vi "Overlay.vi"(0 "Image":T2, 5 "FullArray":dbl[][](array[numeric]), 7 "SelectedGoalSubarray":dbl[](array[numeric]), 9 "ProjectedPosition":cluster{dbl, dbl}, 11 "Enabled Overlay":T1, 13 "encoder":dbl) -> (4 "ImageOut":T2(plugin-control))   [LabVIEW 2012]
uses:
  <vilib>/vision/Image Controls.llb/IMAQ Image.ctl
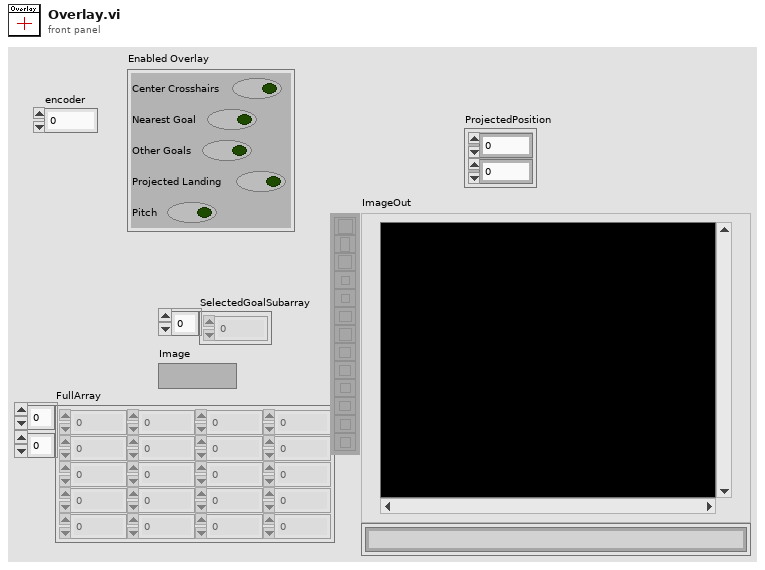
[diagram p1: front panel]
types:
  T1 = cluster{"Center Crosshairs":bool, "Nearest Goal":bool, "Other Goals":bool, "Projected Landing":bool, "Pitch":bool}
  T2 = typedef "IMAQ Image.ctl" = refnum<image>
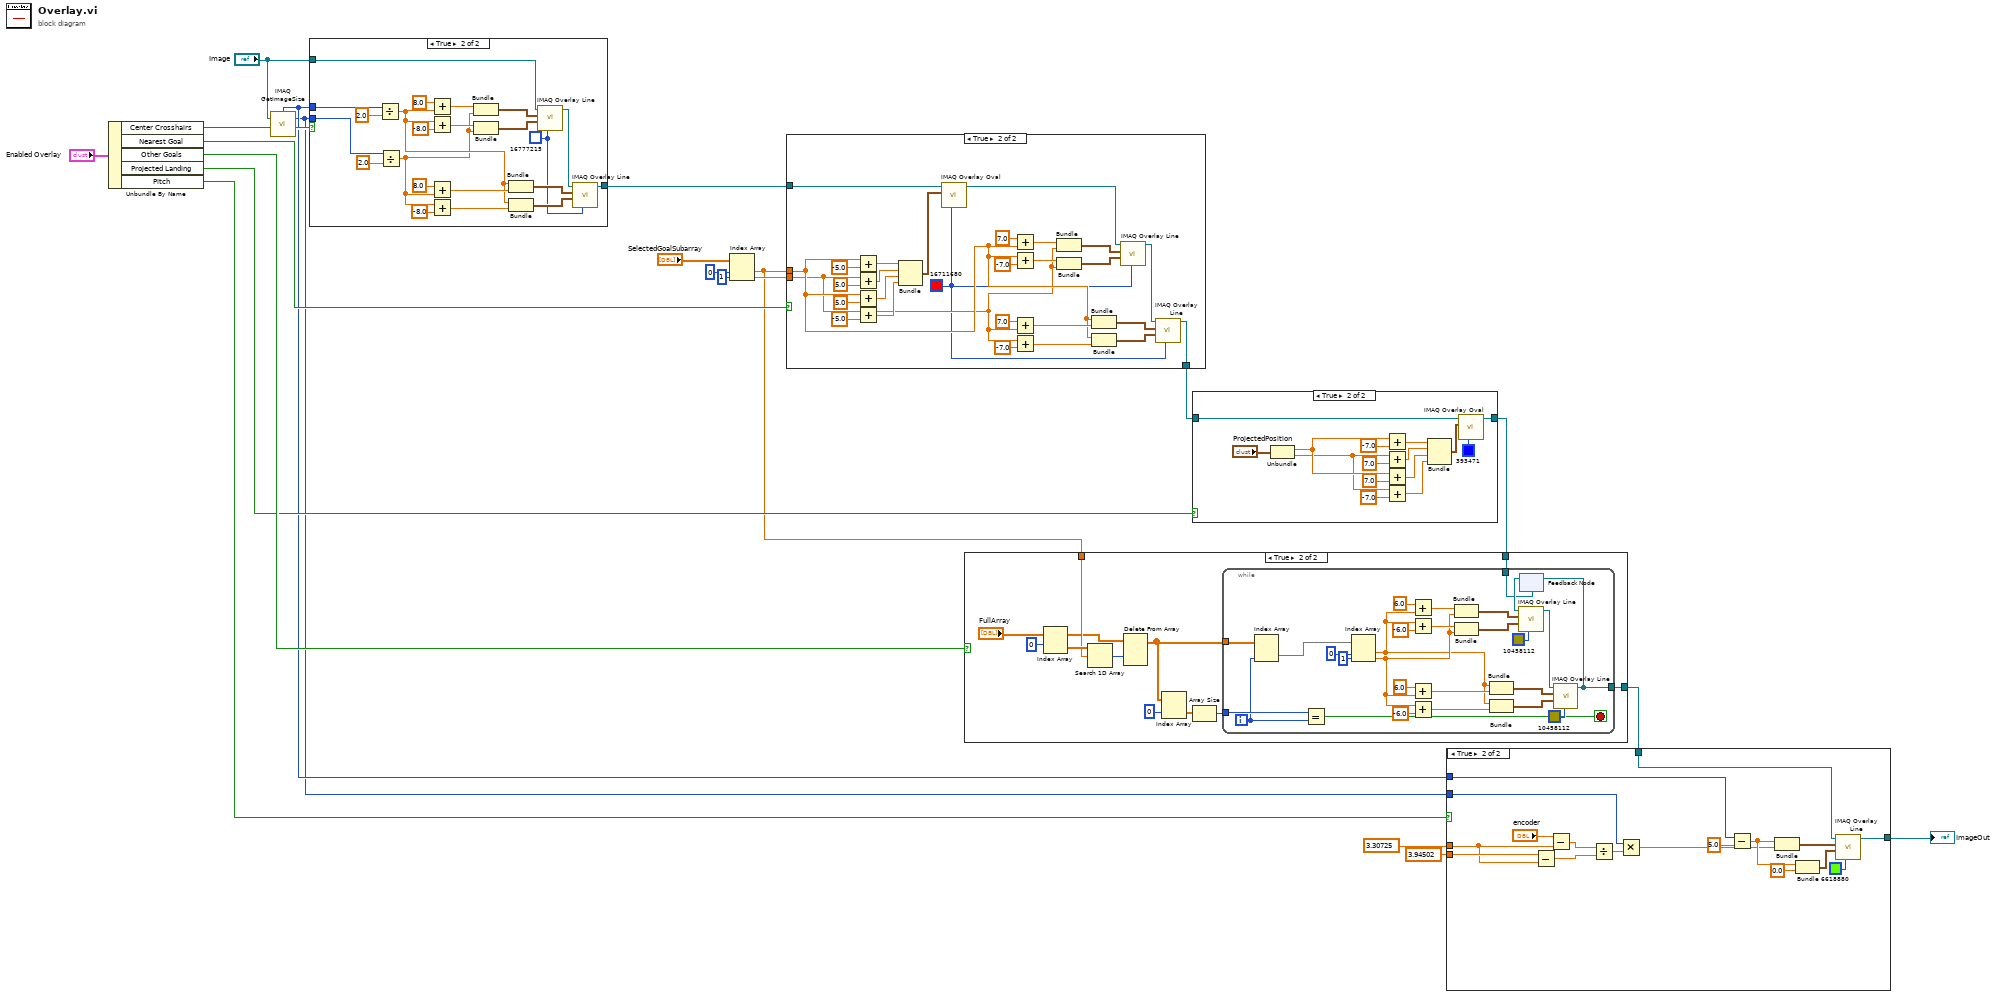
[diagram p0: block diagram]
diagram:
  n1 = Unbundle By Name("Enabled Overlay") -> ("Center Crosshairs"=w15:bool, "Nearest Goal"=w14:bool, "Other Goals"=w13:bool, "Projected Landing"=w12:bool, "Pitch"=w3:bool)
  n2 = call "IMAQ GetImageSize"("Image"="Image") -> ("Y Resolution"=w5:i32, "X Resolution"=w6:i32)  [unwired: 3 in, 1 out]
  n3 = case shown="True" w15 {
    tunnel: [w22 w27] -> w16
    tunnel: "Image" -> [w22 w25]
    tunnel: w5 -> [_ w24]
    tunnel: w6 -> [_ w23]
    frame False {
    }
    frame True {
      w26 = u32 16777215 ("Color")
      n4 = Divide(x=w23, y=2.0) -> (x/y=w29:dbl)
      n5 = Divide(x=w24, y=2.0) -> (x/y=w28:dbl)
      n6 = Add(x=8.0, y=w29) -> (x+y=w39:dbl)
      n7 = Add(x=w29, y=-8.0) -> (x+y=w40:dbl)
      n8 = Add(x=8.0, y=w28) -> (x+y=w34:dbl)
      n9 = Add(x=w28, y=-8.0) -> (x+y=w33:dbl)
      n10 = Bundle(w39, w28) -> (w38:cluster{dbl, dbl})  [unwired: 1 in]
      n11 = Bundle(w40, w28) -> (w37:cluster{dbl, dbl})  [unwired: 1 in]
      n12 = Bundle(w29, w34) -> (w36:cluster{dbl, dbl})  [unwired: 1 in]
      n13 = Bundle(w29, w33) -> (w35:cluster{dbl, dbl})  [unwired: 1 in]
      n14 = call "IMAQ Overlay Line"("Color"=w26, "End Point"=w37, "Start Point"=w38, "Image"=w25) -> ("Image Out"=w32:T2)  [unwired: 6 in, 1 out]
      n15 = call "IMAQ Overlay Line"("Color"=w26, "End Point"=w35, "Start Point"=w36, "Image"=w32) -> ("Image Out"=w27:T2)  [unwired: 6 in, 1 out]
    }
  }
  n16 = Index Array(array="SelectedGoalSubarray", index #1=0 ("index"), index #2=1 ("index")) -> (element #1=w9:dbl, element #2=w18:dbl)
  n17 = case shown="True" w14 {
    tunnel: w9 -> [_ w51]
    tunnel: w18 -> [_ w50]
    tunnel: [w45 w48] -> w11
    tunnel: w16 -> [w45 w46]
    frame False {
    }
    frame True {
      w47 = u32 16711680 ("Color")
      n18 = Add(x=w51, y=-5.0) -> (x+y=w70:dbl)
      n19 = Add(x=w50, y=5.0) -> (x+y=w71:dbl)
      n20 = Add(x=w51, y=5.0) -> (x+y=w69:dbl)
      n21 = Add(x=w50, y=-5.0) -> (x+y=w66:dbl)
      n22 = Bundle(w70, w71, w69, w66) -> (w65:cluster{dbl, dbl, dbl, dbl})  [unwired: 1 in]
      n23 = call "IMAQ Overlay Oval"("Color"=w47, "Bounding Rectangle"=w65, "Image"=w46) -> ("Image Out"=w49:T2)  [unwired: 7 in, 1 out]
      n24 = Add(x=7.0, y=w51) -> (x+y=w59:dbl)
      n25 = Add(x=w51, y=-7.0) -> (x+y=w60:dbl)
      n26 = Add(x=7.0, y=w50) -> (x+y=w54:dbl)
      n27 = Add(x=w50, y=-7.0) -> (x+y=w53:dbl)
      n28 = Bundle(w59, "Numeric"=w50) -> (w58:cluster{dbl, "Numeric":dbl})  [unwired: 1 in]
      n29 = Bundle(w60, "Numeric"=w50) -> (w57:cluster{dbl, "Numeric":dbl})  [unwired: 1 in]
      n30 = Bundle("Numeric"=w51, w54) -> (w56:cluster{"Numeric":dbl, dbl})  [unwired: 1 in]
      n31 = Bundle("Numeric"=w51, w53) -> (w55:cluster{"Numeric":dbl, dbl})  [unwired: 1 in]
      n32 = call "IMAQ Overlay Line"("Color"=w47, "End Point"=w57, "Start Point"=w58, "Image"=w49) -> ("Image Out"=w52:T2)  [unwired: 6 in, 1 out]
      n33 = call "IMAQ Overlay Line"("Color"=w47, "End Point"=w55, "Start Point"=w56, "Image"=w52) -> ("Image Out"=w48:T2)  [unwired: 6 in, 1 out]
    }
  }
  n34 = case shown="True" w12 {
    tunnel: [w74 w80] -> w10
    tunnel: w11 -> [w74 w81]
    frame False {
    }
    frame True {
      n35 = Unbundle("ProjectedPosition") -> (w77:dbl, w76:dbl)
      n36 = Add(x=w77, y=-7.0) -> (x+y=w86:dbl)
      n37 = Add(x=w76, y=7.0) -> (x+y=w87:dbl)
      n38 = Add(x=w77, y=7.0) -> (x+y=w85:dbl)
      n39 = Add(x=w76, y=-7.0) -> (x+y=w82:dbl)
      n40 = Bundle(w86, w87, w85, w82) -> (w78:cluster{dbl, dbl, dbl, dbl})  [unwired: 1 in]
      n41 = call "IMAQ Overlay Oval"("Color"=u32 393471, "Bounding Rectangle"=w78, "Image"=w81) -> ("Image Out"=w80:T2)  [unwired: 7 in, 1 out]
    }
  }
  n42 = case shown="True" w13 {
    tunnel: [w90 w99] -> w7
    tunnel: w10 -> [w90 w98]
    tunnel: w9 -> [_ w97]
    frame False {
    }
    frame True {
      n43 = Index Array(array="FullArray", index (row)=0) -> (element=w101:dbl[])  [unwired: 1 in]
      n44 = Search 1D Array(1D array=w101, element=w97) -> (index of element=w96:i32)  [unwired: 1 in]
      n45 = Delete From Array(array="FullArray", index (row)=w96) -> (array with subset deleted=w93:dbl[][])  [unwired: 2 in, 1 out]
      n46 = Index Array(array=w93, index (row)=0) -> (element=w94:dbl[])  [unwired: 1 in]
      n47 = Array Size(array=w94) -> (size(s)=w92:i32)
      n48 = while {
        tunnel: w93 -> [w106]
        tunnel: [w109] -> w99
        tunnel: w98 -> [w107]
        tunnel: w92 -> [w104]
        i -> [w103]
        stop <- w102 stop-if-true
        n49 = Index Array(array=w106, index (col)=w103) -> (element=w105:dbl[])  [unwired: 1 in]
        n50 = Equal?(x=w104, y=w103) -> (x = y?=w102:bool)
        n51 = Index Array(array=w105, index #1=0 ("index"), index #2=1 ("index")) -> (element #1=w111:dbl, element #2=w120:dbl)
        n52 = Add(x=6.0, y=w111) -> (x+y=w121:dbl)
        n53 = Add(x=w111, y=-6.0) -> (x+y=w122:dbl)
        n54 = Add(x=6.0, y=w120) -> (x+y=w114:dbl)
        n55 = Add(x=w120, y=-6.0) -> (x+y=w113:dbl)
        n56 = Bundle(w121, "Numeric"=w120) -> (w119:cluster{dbl, "Numeric":dbl})  [unwired: 1 in]
        n57 = Bundle(w122, "Numeric"=w120) -> (w118:cluster{dbl, "Numeric":dbl})  [unwired: 1 in]
        n58 = Bundle("Numeric"=w111, w114) -> (w116:cluster{"Numeric":dbl, dbl})  [unwired: 1 in]
        n59 = Bundle("Numeric"=w111, w113) -> (w115:cluster{"Numeric":dbl, dbl})  [unwired: 1 in]
        n60 = feedback #1(w107) -> (w110:T2)
        n61 = call "IMAQ Overlay Line"("Color"=u32 10458112, "End Point"=w118, "Start Point"=w119, "Image"=w110) -> ("Image Out"=w112:T2)  [unwired: 6 in, 1 out]
        n62 = call "IMAQ Overlay Line"("Color"=u32 10458112, "End Point"=w115, "Start Point"=w116, "Image"=w112) -> ("Image Out"=w109:T2)  [unwired: 6 in, 1 out]
        n63 = feedback-in #1(w109) -> ()
      }
    }
  }
  n64 = case shown="True" w3 {
    tunnel: w7 -> [w129 w144]
    tunnel: w6 -> [_ w140]
    tunnel: w5 -> [_ w138]
    tunnel: [w129 w146] -> w4
    tunnel: 3.30725 ("Min") -> [_ w132]
    tunnel: 3.94502 ("Max") -> [_ w133]
    frame False {
    }
    frame True {
      n65 = Subtract(x=w133, y=w132) -> (x-y=w131:dbl)
      n66 = Subtract(x="encoder", y=w132) -> (x-y=w135:dbl)
      n67 = Divide(x=w135, y=w131) -> (x/y=w134:dbl)
      n68 = Multiply(x=w138, y=w134) -> (x*y=w137:dbl)
      n69 = Subtract(x=w140, y=5.0) -> (x-y=w139:dbl)
      n70 = Bundle(w139, w137) -> (w141:cluster{dbl, dbl})  [unwired: 1 in]
      n71 = Bundle(w139, "y"=0.0) -> (w142:cluster{dbl, "y":dbl})  [unwired: 1 in]
      n72 = call "IMAQ Overlay Line"("Color"=u32 6618880, "End Point"=w142, "Start Point"=w141, "Image"=w144) -> ("Image Out"=w146:T2)  [unwired: 6 in, 1 out]
    }
  }
  "ImageOut" <- w4
